vi "DAQmx 9472 8ch Digital Output (SubVI).vi"(0 "9472 Name":tag="9485", 7 "Output Control":bool[](array[boolean])=[FALSE, FALSE, FALSE, FALSE, FALSE, FALSE, FALSE, FALSE], 11 "Error Input":errorcluster, 13 "Stop Program":bool) -> (15 "9472 Error":errorcluster)   [LabVIEW 2012]
uses:
  <vilib>/DAQmx/write.llb/DAQmx Write (Digital 1D Bool NChan 1Samp 1Line).vi
  <vilib>/DAQmx/create/channels.llb/DAQmx Create Channel (DO-Digital Output).vi
  <vilib>/DAQmx/miscellaneous.llb/DAQmx Fill In Error Info.vi
panel:
  # "DAQmx - 9472\n8ch Digital Output\nCreated by Blake Otting \nLast Update 11-20-2012"
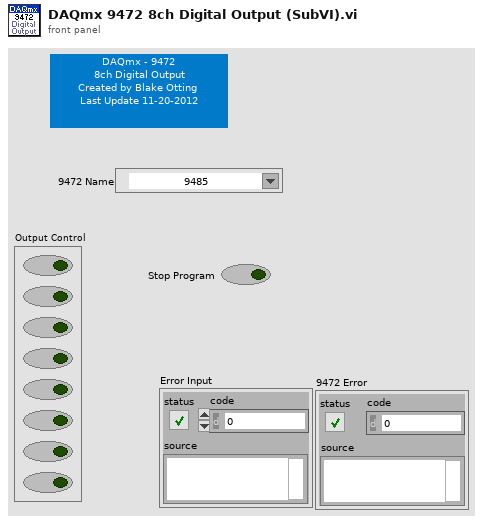
[diagram p1: front panel]
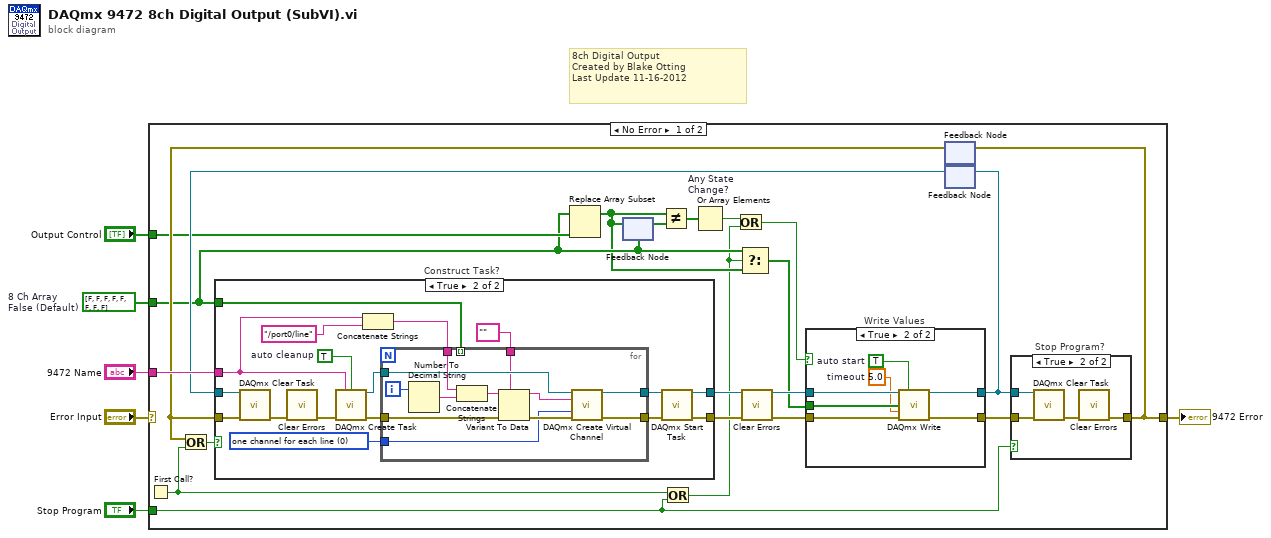
[diagram p0: block diagram]
diagram:
  w3 = bool[] [FALSE, FALSE, FALSE, FALSE, FALSE, FALSE, FALSE, FALSE]  # 8 Ch Array False (Default)
  # "8ch Digital Output\nCreated by Blake Otting \nLast Update 11-16-2012"
  n1 = case shown="No Error" "Error Input" {
    selector: "Error Input" -> [_ w73]
    tunnel: "Output Control" -> [w17 _]
    tunnel: [w25 w73] -> w2
    tunnel: "9472 Name" -> [w26 _]
    tunnel: "Stop Program" -> [w10 _]
    tunnel: w3 -> [w14 _]
    frame No Error {
      n2 = First Call?() -> (First Call?: T/F=w11:bool)
      n3 = Replace Array Subset(array=w14, new element=w17) -> (w13:bool[])  [unwired: 1 in]
      n4 = feedback-in #1(w13) -> ()
      n5 = feedback #1(w14) -> (w16:bool[])
      n6 = Not Equal?(x=w13, y=w16) -> (x != y?=w15:bool[])
      n7 = Or(x=w11, y=w10) -> (x .or. y?=w8:bool)
      n8 = Or Array Elements "Any State\nChange?"(Boolean array=w15) -> (logical OR=w9:bool)
      n9 = Or(x=w9, y=w8) -> (x .or. y?=w7:bool)
      n10 = Select(t=w14, s=w8, f=w13) -> (s? t:f=w12:bool[])
      n11 = feedback #2() -> (w18:errorcluster)  [unwired: 1 in]
      n12 = Or(x=w18, y=w11) -> (x .or. y?=w19:bool)
      n13 = feedback #3() -> (w23:refnum<k21>)  [unwired: 1 in]
      n14 = case "Construct Task?" shown="True" w19 {
        tunnel: [w38 w46] -> w22
        tunnel: [w37 w45] -> w21
        tunnel: w18 -> [w37 w50]
        tunnel: w23 -> [w38 w51]
        tunnel: w26 -> [_ w41]
        tunnel: w14 -> [_ w39]
        frame False {
        }
        frame True {
          w54 = 0 items=["one channel for each line", "one channel for all lines"]
          w55 = TRUE  # auto cleanup
          n15 = call <vilib>:"DAQmx Clear Task.vi"("task in"=w51, "error in"=w50) -> ("error out"=w49:errorcluster)  [unwired: 13 in]
          n16 = call <vilib>:"Clear Errors.vi"("error in (no error)"=w49) -> ("error out"=w48:errorcluster)  [unwired: 6 in]
          n17 = call <vilib>:"DAQmx Create Task.vi"("new task name"=w41, "auto cleanup"=w55, "error in"=w48) -> ("task out"=w52:refnum<k21>, "error out"=w53:errorcluster)  [unwired: 11 in]
          n18 = Concatenate Strings(w41, "/port0/line" ("string")) -> (w44:string)
          n19 = for {
            tunnel: w44 -> [w65]
            tunnel: w53 -> [w64]
            tunnel: [w58] -> w42
            tunnel: w52 -> [w60]
            tunnel: [w59] -> w43
            tunnel: w54 -> [w57]
            tunnel: tag "" ("physical channels") -> [w56]
            tunnel: w39 -> [_] mode=indexing
            i -> [w66]
            n20 = Number To Decimal String(number=w66) -> (decimal integer string=w67:string)  [unwired: 1 in]
            n21 = Concatenate Strings(w65, w67) -> (w61:string)
            n22 = Variant To Data(error in=w64, type=w56, Variant=w61) -> (data=w62:tag, error out=w63:errorcluster)
            n23 = call-poly <vilib>:"DAQmx Create Virtual Channel.vi"("task in"=w60, "lines"=w62, "line grouping"=w57, "error in"=w63) -> ("task out"=w59:refnum<k21>, "error out"=w58:errorcluster)  [unwired: 10 in]
          }
          n24 = call <vilib>:"DAQmx Start Task.vi"("task/channels in"=w43, "error in"=w42) -> ("task out"=w46:refnum<k21>, "error out"=w45:errorcluster)  [unwired: 12 in]
        }
      }
      n25 = call <vilib>:"Clear Errors.vi"("error in (no error)"=w21) -> ("error out"=w20:errorcluster)  [unwired: 6 in]
      n26 = case "Write Values" shown="True" w7 {
        tunnel: w22 -> [w29 w35]
        tunnel: w20 -> [w28 w34]
        tunnel: w12 -> [_ w33]
        tunnel: [w28 w32] -> w27
        tunnel: [w29 w30] -> w24
        frame False {
        }
        frame True {
          w31 = 5.0  # timeout
          w36 = TRUE  # auto start
          n27 = call-poly <vilib>:"DAQmx Write.vi"("task/channels in"=w35, "auto start"=w36, "data"=w33, "timeout"=w31, "error in"=w34) -> ("task out"=w30:refnum<k21>, "error out"=w32:errorcluster)  [unwired: 8 in, 1 out]
        }
      }
      n28 = feedback-in #3(w24) -> ()
      n29 = case "Stop Program?" shown="True" w10 {
        tunnel: w24 -> [_ w70]
        tunnel: w27 -> [w68 w71]
        tunnel: [w68 w69] -> w25
        frame False {
        }
        frame True {
          n30 = call <vilib>:"DAQmx Clear Task.vi"("task in"=w70, "error in"=w71) -> ("error out"=w72:errorcluster)  [unwired: 13 in]
          n31 = call <vilib>:"Clear Errors.vi"("error in (no error)"=w72) -> ("error out"=w69:errorcluster)  [unwired: 6 in]
        }
      }
      n32 = feedback-in #2(w25) -> ()
    }
    frame Error {
    }
  }
  "9472 Error" <- w2
